vi "Animated 1.vi"() -> ()   [LabVIEW 2014, in "Arduino TFT.lvlib"]
uses:
  <vilib>/Aledyne-TSXperts/Arduino Compatible Compiler for LabVIEW/addons/Arduino TFT/Arduino TFT.lvlib
  <vilib>/Aledyne-TSXperts/Arduino Compatible Compiler for LabVIEW/Arduino Compatible Compiler for LabVIEW.lvlib
panel:
  in  "Error In":errorcluster
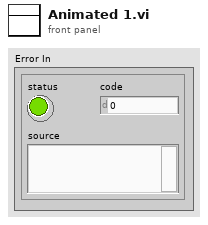
[diagram p1: front panel]
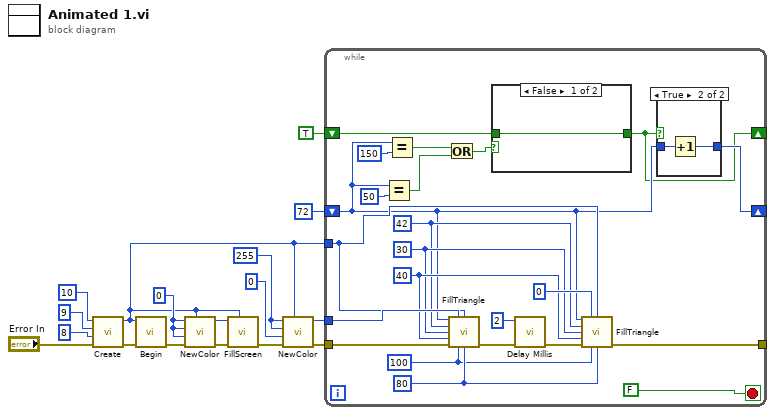
[diagram p0: block diagram]
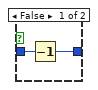
[diagram p2: hidden frame]
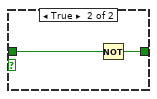
[diagram p3: hidden frame]
diagram:
  w7 = u8 255 ("red")
  w12 = u8 0 ("red")
  n1 = call <vilib>:"Create.vi"("Error In"="Error In", "rst"=u8 8 ("cs"), "rs"=u8 9 ("cs"), "cs"=u8 10) -> ("Error Out"=w13:errorcluster, "Instance"=w4:u32)  [unwired: 4 in]
  n2 = call <vilib>:"Begin.vi"("Error In"=w13, "Instance"=w4) -> ("Error Out"=w11:errorcluster)  [unwired: 8 in]
  n3 = call <vilib>:"NewColor.vi"("Instance"=w4, "Error In"=w11, "blue"=w12, "green"=w12, "red"=w12) -> ("Error Out"=w10:errorcluster, "color"=w9:u16)  [unwired: 5 in]
  n4 = call <vilib>:"FillScreen.vi"("Instance"=w4, "Error In"=w10, "color"=w9) -> ("Error Out"=w8:errorcluster)  [unwired: 8 in]
  n5 = call <vilib>:"NewColor.vi"("Instance"=w4, "Error In"=w8, "blue"=u8 0 ("red"), "green"=w7, "red"=w7) -> ("Error Out"=w2:errorcluster, "color"=w3:u16)  [unwired: 5 in]
  n6 = while {
    shift-right: [w19] -> _
    shift-left: i16 72 ("x") -> [w20]
    tunnel: w4 -> [w28]
    tunnel: w3 -> [w39]
    tunnel: w2 -> [w38]
    tunnel: [w27] -> _
    shift-right: [w18] -> _
    shift-left: TRUE -> [w25]
    stop <- FALSE stop-if-true
    w29 = i16 42 ("x")
    w33 = i16 80 ("x")
    w32 = i16 100 ("x")
    w31 = i16 40 ("x")
    w30 = i16 30 ("x")
    n7 = Equal?(x=w20, y=i16 50) -> (x = y?=w21:bool)
    n8 = Equal?(x=w20, y=i16 150) -> (x = y?=w22:bool)
    n9 = Or(x=w22, y=w21) -> (x .or. y?=w23:bool)
    n10 = call <vilib>:"FillTriangle.vi"("x"=w20, "color"=w39, "Instance"=w28, "y"=w29, "x2"=w30, "y2"=w31, "Error In"=w38, "x3"=w32, "y3"=w33) -> ("Error Out"=w37:errorcluster)  [unwired: 6 in]
    n11 = case shown="False" w23 {
      tunnel: w25 -> [w45 w47]
      tunnel: [w45 w46] -> w18
      frame False {
      }
      frame True {
        n12 = Not(x=w47) -> (.not. x?=w46:bool)
      }
    }
    n13 = call <vilib>:"Delay Millis.vi"("error in (no error)"=w37, "delay"=u32 2) -> ("error out"=w34:errorcluster)  [unwired: 9 in]
    n14 = call <vilib>:"FillTriangle.vi"("x"=w20, "color"=u16 0, "Instance"=w28, "y"=w29, "x2"=w30, "y2"=w31, "Error In"=w34, "x3"=w32, "y3"=w33) -> ("Error Out"=w27:errorcluster)  [unwired: 6 in]
    n15 = case shown="True" w18 {
      tunnel: w20 -> [w41 w44]
      tunnel: [w42 w43] -> w19
      frame False {
        n16 = Decrement(x=w41) -> (x-1=w42:i16)
      }
      frame True {
        n17 = Increment(x=w44) -> (x+1=w43:i16)
      }
    }
  }
